vi "Preview.vi"(8 "error in (no error)":errorcluster, 11 "Scheduler in":refnum<class "Scheduler.lvclass">) -> (0 "error out":errorcluster, 3 "Scheduler out":refnum<class "Scheduler.lvclass">)   [LabVIEW 2020, in "Scheduler.lvlib" / "Scheduler.lvclass"]
uses:
  Scheduler.lvclass
  C:/Users/marco/Documents/GitHub_Lab/TALOS/talos/Father of all uServices/Father of all uServices/Father of all uServices.lvclass
  Run Utilities/Schedule/Array of Runs - GUI.ctl
  Run Utilities/Cell/Cell - GUI.ctl
  Run Utilities/Run Instance/Run Instance - GUI.ctl
  Run Utilities/TypeDefs/Synchronize FPGA Cluster.ctl
  Scheduler.lvclass/Scheduler.ctl
  Scheduler Consumer Case Selector.ctl
  Guardian/Guardian/Requests.ctl
  Father of all uServices/Father of all uServices Messages/Consumer Msg/Consumer Msg.lvclass/Consumer Msg.ctl
  Ancestor/Ancestor/Ancestor.lvclass/Ancestor.ctl
  Guardian/Guardian Messages/Requests from uServices Msg/Requests from uServices Msg.lvclass/Requests from uServices Msg.ctl
  Father of all uServices/Father of all uServices Messages/Consumer Msg/Send Consumer.vi
  Guardian/Guardian Messages/Requests from uServices Msg/Send Requests from uServices.vi
  Support VIs/Generate Error.vi
  FGV/Error Memory/Get Error Description.vi
  Support VIs/Get PC name.vi
  Ancestor/Ancestor/Read ID.vi
  Support VIs/Get Class Name.vi
  <vilib>/Utility/error.llb/Clear Errors.vi
  FGV/Error Memory/Error Memory Core.vi
  <vilib>/AdvancedString/Delimited String to 1D String Array.vi
  Support VIs/Circus Root Path.vi
  FGV/Error Memory/Error Crt Lvl checker.vi
  FGV/Error Memory/Error Memory Core.vi/40c8088d-b597-4017-91af-faa98e00292e.vi
  FGV/Error Memory/Error Memory Core.vi/d4a3ab98-063c-4e44-b43d-fbdcfe6c2be2.vi
  Father of all uServices/Father of all uServices/Father of all uServices.lvclass
  C:/Users/marco/Documents/GitHub_Lab/TALOS/builds/Actor Framework PPL/Actor Framework.lvlibp/1abvi3w/vi.lib/ActorFramework/Actor/Actor.lvclass
  Father of all uServices/Father of all uServices/Children Methods/Get GUI Item Value - Variant.vi
  Support VIs/Global Constants.vi
  builds/Actor Framework PPL/Actor Framework.lvlibp/1abvi3w/vi.lib/ActorFramework/Actor/Read Self Enqueuer.vi
  <userlib>/_OpenG.lib/lvdata/lvdata.llb/Get Strings from Enum__ogtk.vi
  builds/Actor Framework PPL/Actor Framework.lvlibp/1abvi3w/vi.lib/ActorFramework/Message Enqueuer/Enqueue.vi
  Support VIs/Global Memory.vi
  <vilib>/Utility/LVClass/Get LV Class Name.vi
  Support VIs/Is in Packed Library.vi
  Support VIs/TALOS Root path.vi
  Support VIs/Read CSV worksheet.vi
  <vilib>/Utility/error.llb/General Error Handler.vi
  Support VIs/Error Log.vi
  builds/Actor Framework PPL/Actor Framework.lvlibp/1abvi3w/vi.lib/ActorFramework/Actor/Read Caller Enqueuer.vi
  Father of all uServices/Father of all uServices Messages/Consumer Msg/Consumer Msg.lvclass
  Ancestor/Ancestor/Ancestor.lvclass
  <vilib>/Comparison/Equal/Equal Functor/Equal Functor.lvclass
  Guardian/Guardian Messages/Requests from uServices Msg/Requests from uServices Msg.lvclass
  Run Utilities/Sequence of SBlocks/Sequence of SBlocks.lvclass
  Run Utilities/Schedule/Schedule.lvclass
  Run Utilities/Run Utilities.lvlib
  Scheduling_gif.vi
  Abort_gif.vi
  C:/Users/marco/Documents/GitHub_Lab/TALOS/talos/Ancestor/Ancestor/Ancestor.lvclass
  TALOS.lvlib
  Guardian/Guardian/Guardian.lvclass
  Run Utilities/Run Instance/Run Instance.lvclass
  Run Utilities/Cell/Schedule Cell.lvclass
panel:
  out "Sync. Mask":T1[](array[typedef])
  in  "ACCEPT":bool
  in  "CANCEL":bool
  out "Prepared Schedules":cluster{"Continuous":bool, "Array of Runs":T2}[](array[cluster]) {"Array of Runs"."Number of cycles" min=1}
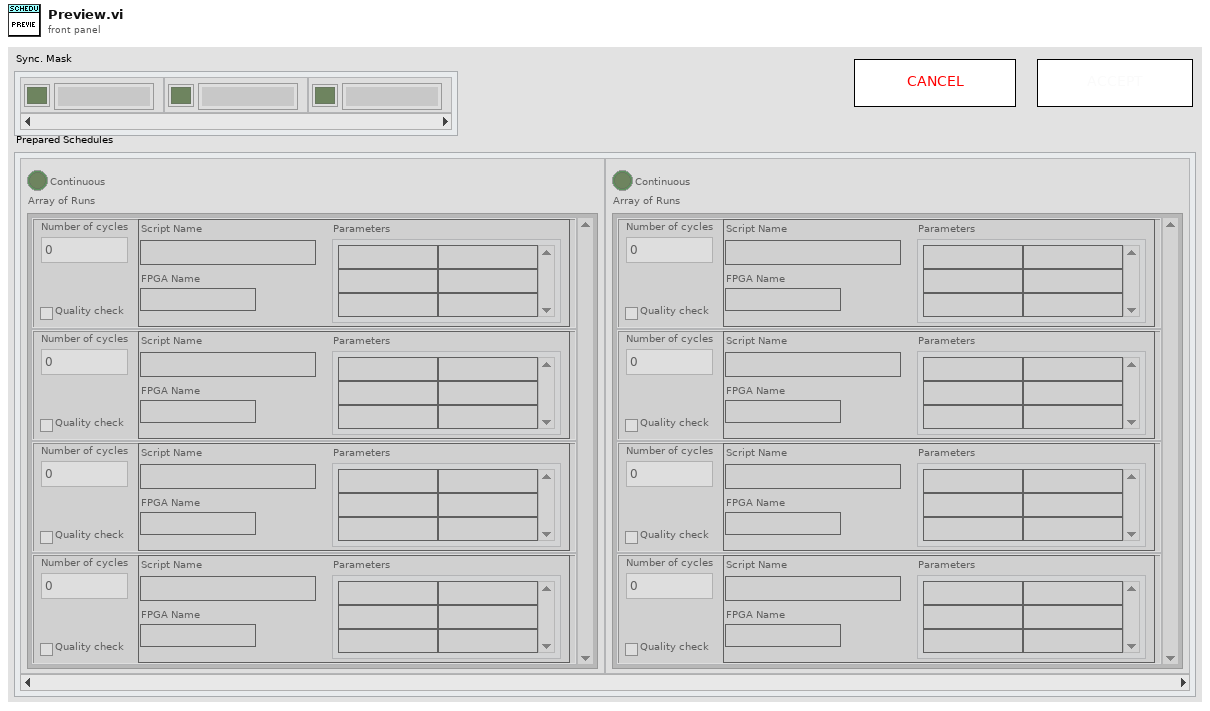
[diagram p1: front panel]
types:
  T1 = typedef "TALOS.lvlib/Run Utilities.lvlib/Synchronize FPGA Cluster.ctl" = cluster{"Status":bool, "FPGA Name":string}
  T2 = typedef "TALOS.lvlib/Run Utilities.lvlib/Schedule.lvclass/Array of Runs - GUI.ctl" = T3[]
  T3 = typedef "TALOS.lvlib/Run Utilities.lvlib/Schedule Cell.lvclass/Cell - GUI.ctl" = cluster{"Background Color":u32, "Number of cycles":u32, "Single RUN":T4, "Quality check":bool, "Cell Type":string}
  T4 = typedef "TALOS.lvlib/Run Utilities.lvlib/Run Instance.lvclass/Run Instance - GUI.ctl" = cluster{"Script Name":string, "Parameters":string[][], "FPGA Name":string}
  T5 = enum8{"Enabled", "Disabled", "Disabled and Grayed Out"}
  T6 = typedef "TALOS.lvlib/Guardian.lvlib/Guardian.lvclass/Requests.ctl" = enum16{"Ready to Launch", "Start RUN", "Stop RUN", "Update DAQ Params", "Update Error Listbox", "Update Run Status", "Update Kasli Log", "Run Stopped with Errors", "Switch uS View"}
  T7 = typedef "Scheduler.lvlib/Scheduler.lvclass/Scheduler Consumer Case Selector.ctl" = enum16{"Add SBlock", "Update GUI", "Move SBlock", "Select SBlock", "Update Cont.", "Load", "Save", "Reset", "Send to Tamer", "Edit SBlock", "Duplicate SBlock", "Delete SBlock", "Update SBlock", "Init", "Split/Combine Schedules", "Reschedule", "Load Parameters"}
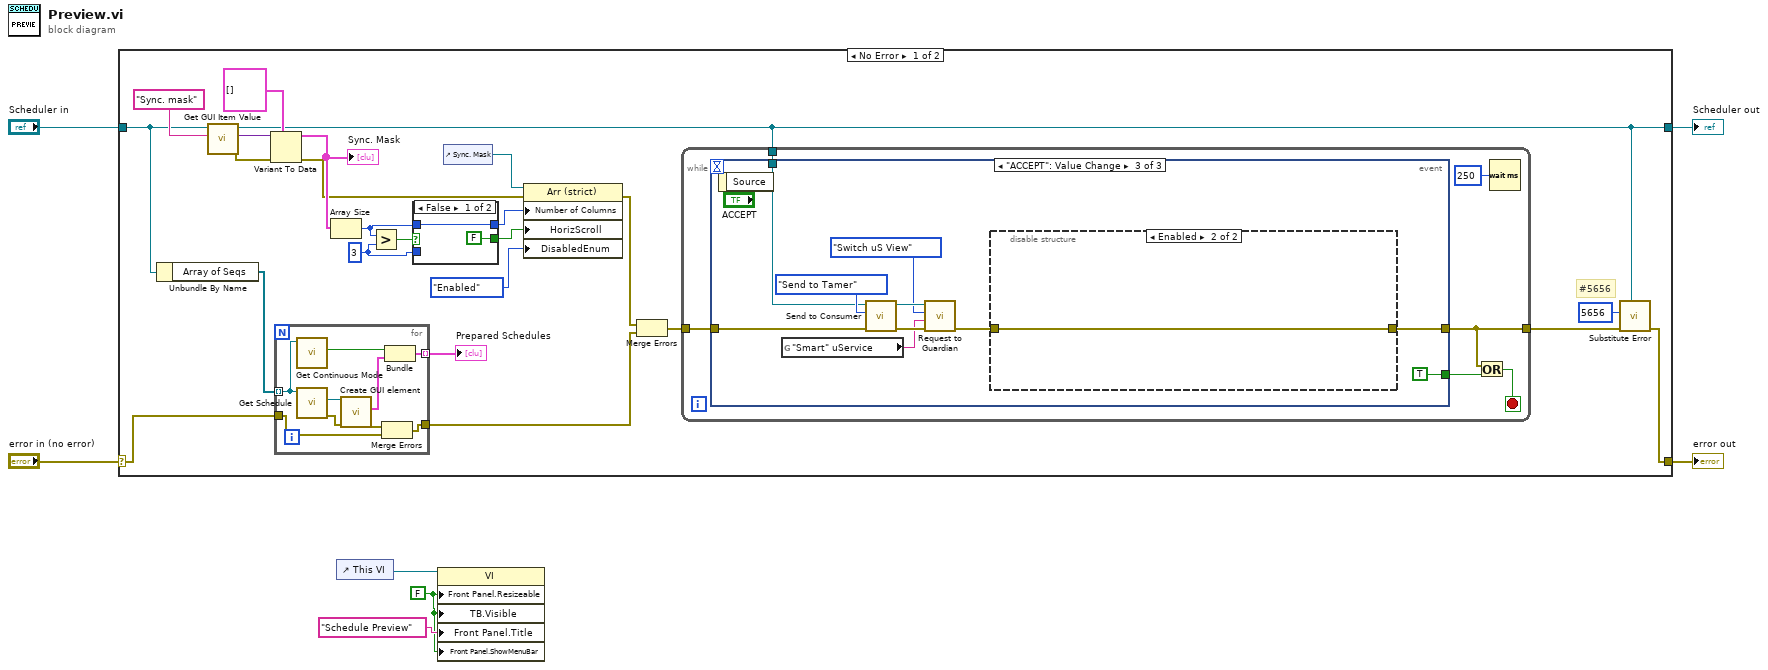
[diagram p0: block diagram]
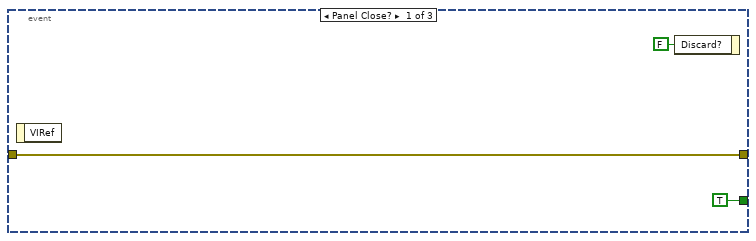
[diagram p2: hidden frame]
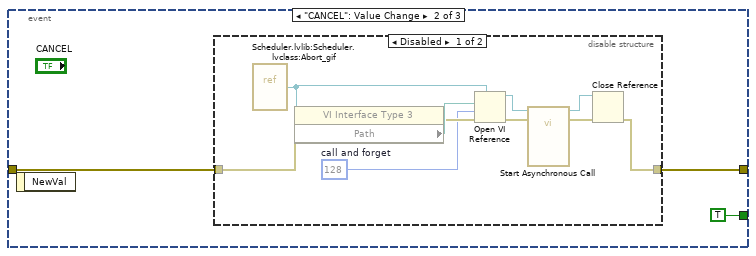
[diagram p3: hidden frame]
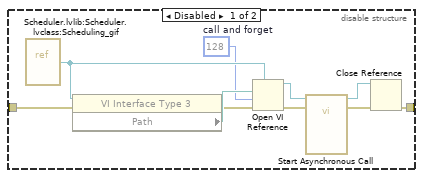
[diagram p5: hidden frame]
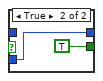
[diagram p6: hidden frame]
diagram:
  w1 = FALSE ("Front Panel Window:Resizable")
  n1 = case shown="No Error" "error in (no error)" {
    selector: "error in (no error)" -> [w30 w90]
    tunnel: [w11 w90] -> w6
    tunnel: [w10 w89] -> w4
    tunnel: "Scheduler in" -> [w8 w89]
    frame No Error {
      w20 = 3 ("y")
      # "#5656"
      n2 = Unbundle By Name(w8) -> ("Array of Seqs"=w31:refnum<class "Sequence of SBlocks.lvclass">[])
      n3 = call-poly "Get GUI Item Value.vi"("FP Item Name"="Sync. mask", "uService Template in"=w8) -> ("error out"=w26:errorcluster, "Value"=w28:variant, "uService Template out"=w10:refnum<class "Scheduler.lvclass">)  [unwired: 7 in]
      n4 = Variant To Data(error in=w26, type=T1[] [], Variant=w28) -> (data=w18:T1[], error out=w16:errorcluster)
      "Sync. Mask" <- w18
      n5 = for {
        tunnel: w31 -> [w84] mode=indexing
        tunnel: w30 -> [w77]
        tunnel: [w80] -> w25 mode=indexing
        tunnel: [w79] -> w14
        n6 = call-dynamic "Get Continuous Mode.vi"("Sequence of SBlocks in"=w84) -> ("Continuous"=w83:bool)  [unwired: 8 in, 2 out]
        n7 = call-dynamic "Get Schedule.vi"("Sequence of SBlocks in"=w84) -> ("error out"=w81:errorcluster, "Schedule"=w76:refnum<class "Schedule.lvclass">)  [unwired: 8 in, 1 out]
        n8 = call-dynamic "Create GUI element.vi"("error in (no error)"=w81, "Schedule in"=w76) -> ("error out"=w78:errorcluster, "Array of Runs"=w82:T2)  [unwired: 7 in, 1 out]
        n9 = Merge Errors(w78, w77) -> (w79:errorcluster)
        n10 = Bundle("Continuous"=w83, "Array of Runs"=w82) -> (w80:cluster{"Continuous":bool, "Array of Runs":T2})  [unwired: 1 in]
      }
      "Prepared Schedules" <- w25
      n11 = Array Size(array=w18) -> (size(s)=w24:i32)
      n12 = Greater?(x=w24, y=w20) -> (0:w21:bool)
      n13 = case shown="False" w21 {
        tunnel: [w85 w87] -> w22
        tunnel: [FALSE TRUE] -> w23
        tunnel: w24 -> [w85 _]
        tunnel: w20 -> [_ w87]
        frame False {
        }
        frame True {
        }
      }
      n14 = control-ref of="Sync. Mask"() -> (w17:refnum<vi>)
      n15 = property class="Arr (strict)"(reference=w17, error in=w16, "Number of Columns"=w22, "HorizScroll"=w23, "DisabledEnum"=T5."Enabled" ("Disabled")) -> (error out=w15:errorcluster)  [unwired: 1 out]
      n16 = Merge Errors(w15, w14) -> (w13:errorcluster)
      n17 = while {
        tunnel: w13 -> [w36]
        tunnel: [w33] -> w12
        tunnel: w10 -> [w32]
        stop <- w35 stop-if-true
        n18 = event shown="[2] \"ACCEPT\": Value Change" {
          selector: _ -> [_ _ _]
          dyn-events: _ -> [_ _ _]
          timeout: _ -> [_ _ _]
          tunnel: w36 -> [w39 w41 w63]
          tunnel: [w39 w42 w61] -> w33
          tunnel: [TRUE TRUE TRUE] -> w34
          tunnel: w32 -> [_ _ w55]
          event Panel Close? {
            n19 = event-data() -> ()  [unwired: 1 in, 1 out]
            n20 = event-data("Discard?"=FALSE) -> ()  [unwired: 1 in, 1 out]
          }
          event "CANCEL": Value Change {
            n21 = event-data() -> ()  [unwired: 1 in, 1 out]
            n22 = disable-structure shown="Disabled" {
              disable-tunnel: [w45 w54] -> w42
              disable-tunnel: w41 -> [w44 w54]
              frame Disabled {
                w46 = 128  # call and forget
                n23 = vi-ref "Scheduler.lvlib:Scheduler.lvclass:Abort_gif.vi"() -> (w52:refnum<vi>)
                n24 = property class="VI Interface Type 3"(reference=w52, error in=w44) -> (error out=w47:errorcluster, "Path"=w48:path)  [unwired: 1 out]
                n25 = Open VI Reference(type specifier VI Refnum (for type only)=w52, vi path=w48, options=w46, error in (no error)=w47) -> (vi reference=w50:refnum<vi>, error out=w53:errorcluster)  [unwired: 2 in]
                n26 = call-by-ref "Start Asynchronous Call"(reference=w50, error in=w53) -> (reference out=w49:refnum<vi>, error out=w51:errorcluster)  [unwired: 12 in]
                n27 = Close Reference(reference=w49, error in (no error)=w51) -> (error out=w45:errorcluster)
              }
              frame Enabled {
              }
            }
          }
          event "ACCEPT": Value Change {
            n28 = event-data() -> ()  [unwired: 1 in, 1 out]
            n29 = global read "Global Constants.vi" "\"Smart\" uService"() -> (w56:string)
            n30 = call "Send to Consumer.vi"("error in (no error)"=w63, "Case ID"=Scheduler_Consumer_Case_Selector."Send to Tamer" ("Shifter Panel Consumer Case Selector"), "uService Template in"=w55) -> ("error out"=w60:errorcluster, "uService Template out"=w58:refnum<class "Scheduler.lvclass">)  [unwired: 7 in]
            n31 = call "Request to Guardian.vi"("error in (no error)"=w60, "Data"=w56, "Requests"=Requests."Switch uS View", "Father of all uServices in"=w58) -> ("error out"=w59:errorcluster)  [unwired: 6 in, 1 out]
            n32 = disable-structure shown="Enabled" {
              disable-tunnel: [w66 w75] -> w61
              disable-tunnel: w59 -> [w65 w75]
              frame Disabled {
                w67 = 128  # call and forget
                n33 = vi-ref "Scheduler.lvlib:Scheduler.lvclass:Scheduling_gif.vi"() -> (w73:refnum<vi>)
                n34 = property class="VI Interface Type 3"(reference=w73, error in=w65) -> (error out=w68:errorcluster, "Path"=w69:path)  [unwired: 1 out]
                n35 = Open VI Reference(type specifier VI Refnum (for type only)=w73, vi path=w69, options=w67, error in (no error)=w68) -> (vi reference=w71:refnum<vi>, error out=w74:errorcluster)  [unwired: 2 in]
                n36 = call-by-ref "Start Asynchronous Call"(reference=w71, error in=w74) -> (reference out=w70:refnum<vi>, error out=w72:errorcluster)  [unwired: 12 in]
                n37 = Close Reference(reference=w70, error in (no error)=w72) -> (error out=w66:errorcluster)
              }
              frame Enabled {
              }
            }
          }
        }
        n38 = Or(x=w33, y=w34) -> (x .or. y?=w35:bool)
        n39 = Wait (ms)(milliseconds to wait=u32 250) -> ()  [unwired: 1 out]
      }
      n40 = call "Substitute Error.vi"("LabVIEW Object"=w10, "error in (no error)"=w12, "Error Code"=5656) -> ("error out"=w11:errorcluster)  [unwired: 8 in]
    }
    frame Error {
    }
  }
  "error out" <- w6
  "Scheduler out" <- w4
  n41 = control-ref of="This VI"() -> (w3:refnum<vi>)
  n42 = property class="VI"(reference=w3, "Front Panel.Resizeable"=w1, "TB.Visible"=w1, "Front Panel.Title"="Schedule Preview" ("Front Panel Window:Title"), "Front Panel.ShowMenuBar"=w1) -> ()  [unwired: 1 in, 2 out]
